vi "Draw 2D Range Data.vi"(7 "draw options":T2={"Background Color"=16777215, "Grid Color"=13816530, "Angle Units"=enum."Degrees", "Draw Solid Background"=TRUE, "Draw Grid"=TRUE, "Grid Spacing"=0.25, "AutoScale"=FALSE, "Fit to Radius"=1.0, "data row options"=[]}, 8 "error in (no error)":errorcluster, 9 "DrawAreaSize":T5={"Width"=100, "Height"=100}, 10 "data":T1, 11 "picture in":picture) -> (0 "error out":errorcluster, 3 "picture out":picture)   [LabVIEW 2017, in "NI_Robotics_2D Rangefinder Picture.lvlib"]
uses:
  <vilib>/robotics/Controls/2D Rangefinder/2D Rangefinder Picture/NI_Robotics_2D Rangefinder Picture.lvlib
  <vilib>/Utility/miscctls.llb/LVBoundsTypeDef.ctl
  <vilib>/robotics/Controls/2D Rangefinder/2D Rangefinder Picture/Draw Options.ctl
  <vilib>/robotics/Controls/Utilities/Angle Units.ctl
  <vilib>/robotics/Controls/2D Rangefinder/2D Rangefinder Picture/Data Row Options.ctl
  <vilib>/robotics/Controls/2D Rangefinder/2D Rangefinder Picture/Rangefinder Data.ctl
  <vilib>/Utility/AngleManip/Degrees to Radians.vi
  <vilib>/Utility/AngleManip/Degrees to Radians (Array DBL).vi
  <vilib>/robotics/Controls/Utilities/NI_Robotics_Control Utilities.lvlib
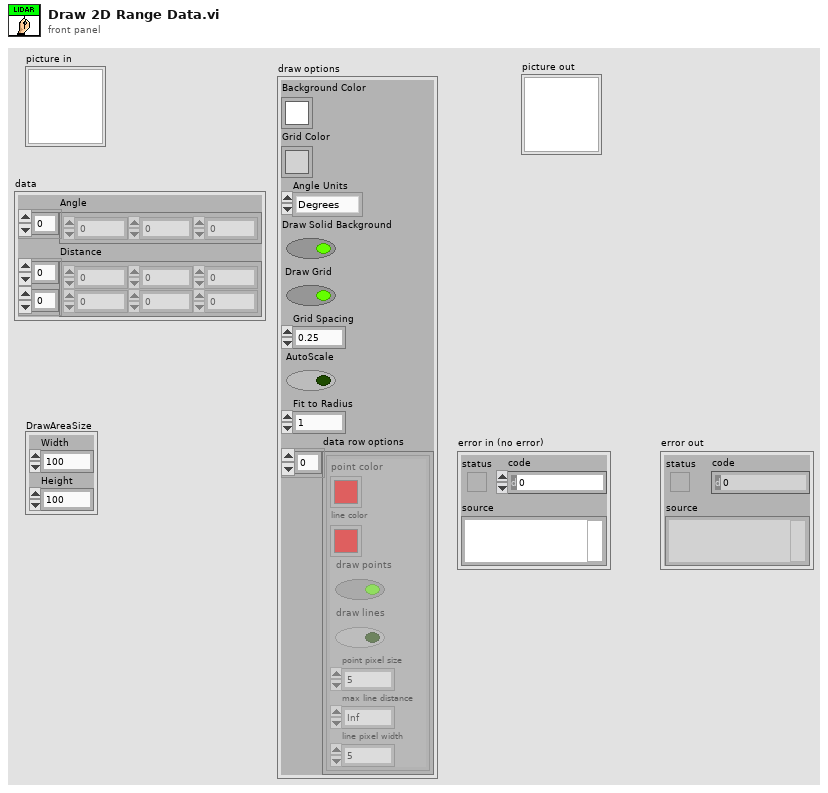
[diagram p1: front panel]
types:
  T1 = typedef "NI_Robotics_2D Rangefinder Picture.lvlib/Rangefinder Data.ctl" = cluster{"Angle":dbl[], "Distance":dbl[][]}
  T2 = typedef "NI_Robotics_2D Rangefinder Picture.lvlib/Draw Options.ctl" = cluster{"Background Color":u32, "Grid Color":u32, "Angle Units":T3, "Draw Solid Background":bool, "Draw Grid":bool, "Grid Spacing":dbl, "AutoScale":bool, "Fit to Radius":dbl, "data row options":T4[]}
  T3 = typedef "NI_Robotics_Control Utilities.lvlib/Angle Units.ctl" = enum16{"Radians", "Degrees"}
  T4 = typedef "NI_Robotics_2D Rangefinder Picture.lvlib/Data Row Options.ctl" = cluster{"point color":u32, "line color":u32, "draw points":bool, "draw lines":bool, "point pixel size":u16, "max line distance":dbl, "line pixel width":u16}
  T5 = typedef "LVBoundsTypeDef.ctl" = cluster{"Width":u32, "Height":u32}
  T6 = typedef "NI_Robotics_2D Rangefinder Picture.lvlib/Cartesian Data.ctl" = cluster{"xy points":cluster{"xy set":cluster{"x":dbl, "y":dbl}[], "distance set":dbl[]}[], "max radius":dbl}
  T7 = typedef "NI_Robotics_2D Rangefinder Picture.lvlib/Scaling Info.ctl" = cluster{"pixels per unit":dbl, "fit radius (units)":dbl, "center point (pixels)":cluster{"x":i16, "y":i16}}
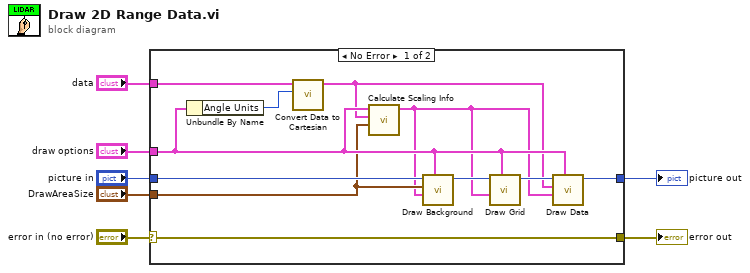
[diagram p0: block diagram]
diagram:
  n1 = case shown="No Error" "error in (no error)" {
    selector: "error in (no error)" -> [w10 w20]
    tunnel: [w10 w20] -> w6
    tunnel: "picture in" -> [w18 w19]
    tunnel: [w13 w19] -> w4
    tunnel: "DrawAreaSize" -> [w9 _]
    tunnel: "draw options" -> [w12 _]
    tunnel: "data" -> [w16 _]
    frame No Error {
      n2 = Unbundle By Name(w12) -> ("Angle Units"=w15:T3)
      n3 = call <vilib>:"Convert Data to Cartesian.vi"("angle units"=w15, "data"=w16) -> ("cartesian data"=w11:T6)  [unwired: 9 in]
      n4 = call <vilib>:"Calculate Scaling Info.vi"("DrawAreaSize"=w9, "cartesian data"=w11, "draw options in"=w12) -> ("scaling info"=w8:T7)  [unwired: 8 in]
      n5 = call <vilib>:"Draw Background.vi"("draw options"=w12, "scaling info"=w8, "DrawAreaSize"=w9, "picture in"=w18) -> ("picture out"=w17:picture)  [unwired: 7 in]
      n6 = call <vilib>:"Draw Grid.vi"("draw options"=w12, "scaling info"=w8, "picture in"=w17) -> ("picture out"=w14:picture)  [unwired: 8 in]
      n7 = call <vilib>:"Draw Data.vi"("draw options"=w12, "scaling info"=w8, "cartesian data"=w11, "picture in"=w14) -> ("picture out"=w13:picture)  [unwired: 7 in]
    }
    frame Error {
    }
  }
  "picture out" <- w4
  "error out" <- w6
